vi "Compile APU 1.4 Data.vi"(8 "error in (no error)":errorcluster, 11 "Device Item Ref in":T3 format="%.0x") -> (0 "error out":errorcluster, 2 "APUs":T1[](array[typedef]), 3 "Device Item Ref out":T3 format="%.0x")   [LabVIEW 2015, in "Engine Simulation Toolkit System Explorer.lvlib"]
uses:
  Engine Simulation Toolkit System Explorer.lvlib
  <vilib>/NI Veristand/Custom Device API/Custom Device Item Ref.ctl
  Shared/1.4 APU Engine Data.ctl
  Shared/1.4 APU Engine FIFO Idxs.ctl
  Shared/Properties.vi
  Shared/Constants and GUIDs.vi
  <vilib>/NI Veristand/Custom Device Tools/Custom Device Utility Library/NI VeriStand - Search for All Items by GUID.vi
  <vilib>/NI Veristand/Custom Device API/Get Item Property (String).vi
  <vilib>/NI Veristand/Custom Device API/Get Item Property (Double).vi
  <vilib>/NI Veristand/Custom Device API/Get Item Property (Boolean).vi
  <vilib>/NI Veristand/Custom Device API/Get Item Property (U16).vi
  <vilib>/NI Veristand/Custom Device Tools/Custom Device Utility Library/NI VeriStand - Search for Item by GUID.vi
  Shared/Engine Simulation Toolkit Shared.lvlib
  <vilib>/NI Veristand/Custom Device API/Custom Device API.lvlib
  <vilib>/NI Veristand/Custom Device Tools/Custom Device Utility Library/Custom Device Utility Library.lvlib
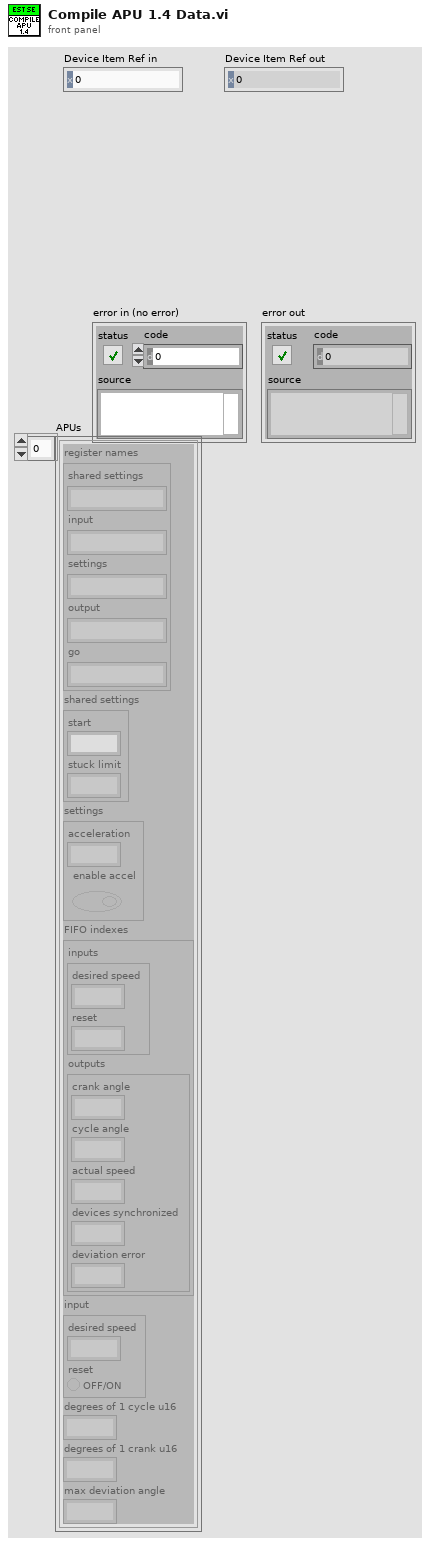
[diagram p1: front panel]
types:
  T1 = typedef "Engine Simulation Toolkit Shared.lvlib/1.4 APU Engine Data.ctl" = cluster{"register names":cluster{"shared settings":string, "input":string, "settings":string, "output":string, "go":string}, "shared settings":cluster{"start":fxp<+,17,17>, "stuck limit":fxp<+,18,18>}, "settings":cluster{"acceleration":fxp<+,18,-20>, "enable accel":bool}, "FIFO indexes":T2, "input":cluster{"desired speed":fxp<+/-,23,2>, "reset":bool}, "degrees of 1 cycle u16":dbl, "degrees of 1 crank u16":dbl, "max deviation angle":dbl}
  T2 = typedef "Engine Simulation Toolkit Shared.lvlib/1.4 APU Engine FIFO Idxs.ctl" = cluster{"inputs":cluster{"desired speed":i32, "reset":i32}, "outputs":cluster{"crank angle":i32, "cycle angle":i32, "actual speed":i32, "devices synchronized":i32, "deviation error":i32}}
  T3 = typedef "Custom Device API.lvlib/Custom Device Item Ref.ctl" = u64
  T4 = typedef "Engine Simulation Toolkit Shared.lvlib/Channel.ctl" = cluster{"Name":string, "Units":string, "Default":dbl, "Description":string, "Scalable":bool}
  T5 = cluster{"desired speed":fxp<+/-,23,2>, "reset":bool}
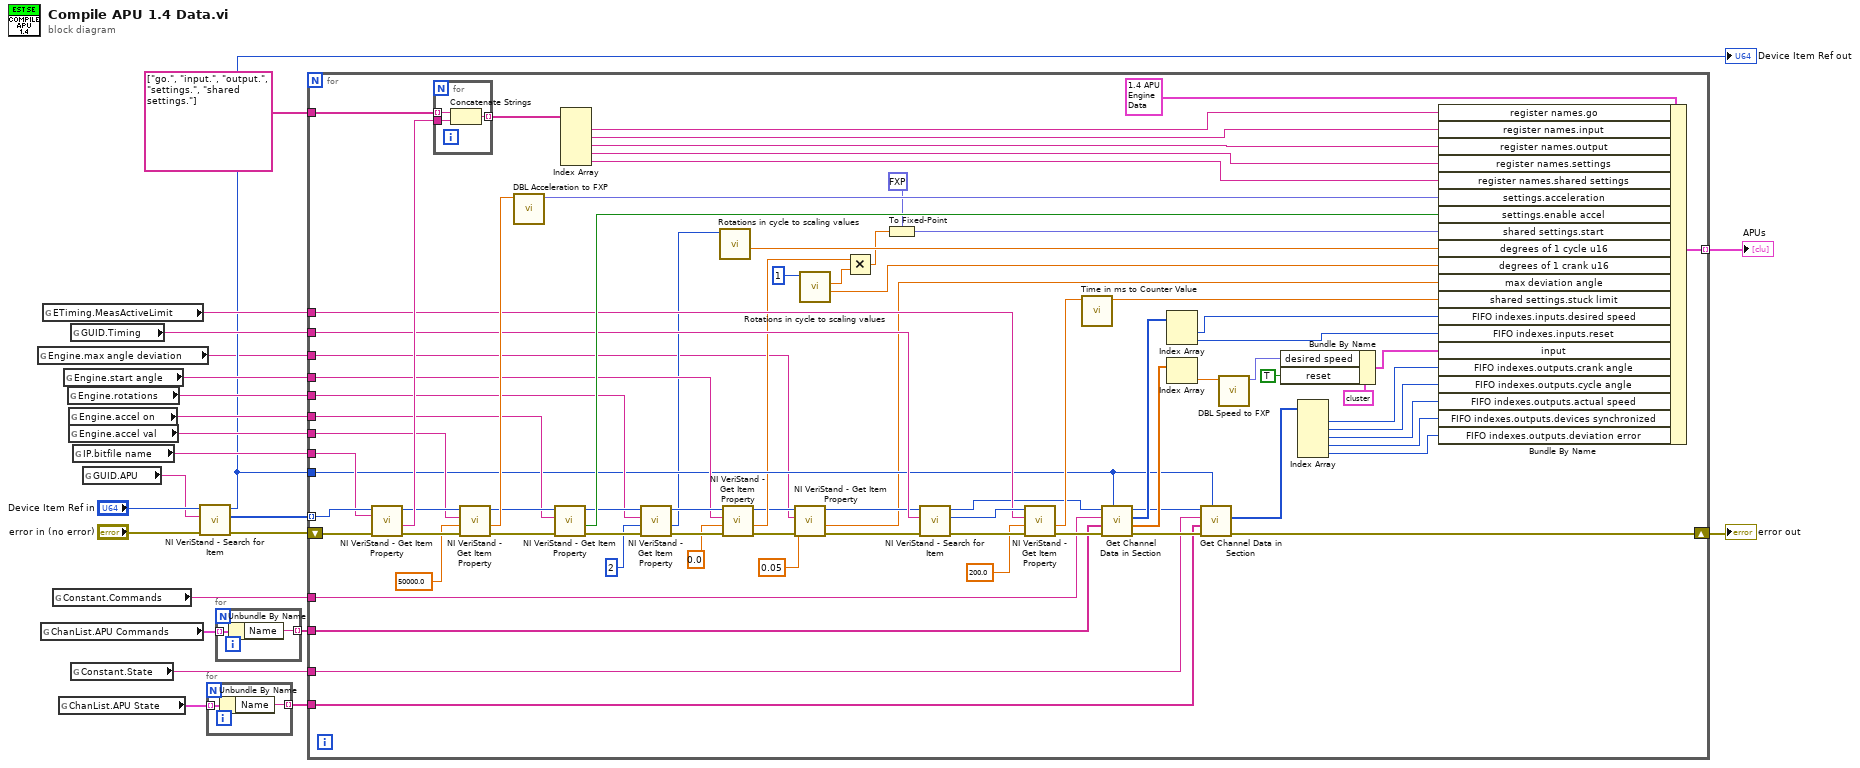
[diagram p0: block diagram]
diagram:
  n1 = global read "Properties.vi" "Engine.max angle deviation"() -> (w1:string)
  n2 = global read "Constants and GUIDs.vi" "ChanList.APU Commands"() -> (w7:T4[])
  n3 = global read "Properties.vi" "ETiming.MeasActiveLimit"() -> (w11:string)
  n4 = global read "Constants and GUIDs.vi" "Constant.Commands"() -> (w10:string)
  n5 = global read "Constants and GUIDs.vi" "ChanList.APU State"() -> (w5:T4[])
  n6 = global read "Properties.vi" "Engine.start angle"() -> (w13:string)
  n7 = global read "Properties.vi" "Engine.rotations"() -> (w14:string)
  n8 = global read "Properties.vi" "Engine.accel on"() -> (w15:string)
  n9 = global read "Properties.vi" "Engine.accel val"() -> (w17:string)
  n10 = global read "Constants and GUIDs.vi" "GUID.Timing"() -> (w12:string)
  n11 = global read "Constants and GUIDs.vi" "Constant.State"() -> (w8:string)
  n12 = global read "Properties.vi" "IP.bitfile name"() -> (w19:string)
  n13 = global read "Constants and GUIDs.vi" "GUID.APU"() -> (w21:string)
  n14 = call-poly <vilib>:"NI VeriStand - Search for Item.vi"("error in"="error in (no error)", "Item GUID"=w21, "Section Ref in"="Device Item Ref in") -> ("error out"=w20:errorcluster, "Item Refs"=w3:T3[], "Section Ref out"=w9:T3)  [unwired: 5 in, 1 out]
  "Device Item Ref out" <- w9
  n15 = for {
    tunnel: w5 -> [w25] mode=indexing
    tunnel: [w24] -> w4 mode=indexing
    n16 = Unbundle By Name(w25) -> ("Name"=w24:string)
  }
  n17 = for {
    tunnel: w7 -> [w27] mode=indexing
    tunnel: [w26] -> w6 mode=indexing
    n18 = Unbundle By Name(w27) -> ("Name"=w26:string)
  }
  n19 = for {
    shift-right: [w62] -> w16
    shift-left: w20 -> [w106]
    tunnel: w3 -> [w105] mode=indexing
    tunnel: w19 -> [w104]
    tunnel: string[] ["go.", "input.", "output.", "settings.", "shared settings."] -> [w102]
    tunnel: w17 -> [w97]
    tunnel: w15 -> [w91]
    tunnel: w14 -> [w87]
    tunnel: w13 -> [w84]
    tunnel: w12 -> [w81]
    tunnel: w11 -> [w78]
    tunnel: w10 -> [w73]
    tunnel: w6 -> [w51]
    tunnel: [w67] -> w2 mode=indexing
    tunnel: w9 -> [w61]
    tunnel: w8 -> [w59]
    tunnel: w4 -> [w50]
    tunnel: w1 -> [w29]
    n20 = call-poly <vilib>:"NI VeriStand - Get Item Property.vi"("error in (no error)"=w106, "Property Name"=w104, "Item Ref in"=w105) -> ("error out"=w98:errorcluster, "Value"=w103:string, "Item Ref out"=w99:T3)  [unwired: 5 in, 1 out]
    n21 = for {
      tunnel: w103 -> [w109]
      tunnel: w102 -> [w108] mode=indexing
      tunnel: [w107] -> w100 mode=indexing
      n22 = Concatenate Strings(w108, w109) -> (w107:string)
    }
    n23 = call-poly <vilib>:"NI VeriStand - Get Item Property.vi"("error in (no error)"=w98, "Default Value"=50000.0, "Property Name"=w97, "Item Ref in"=w99) -> ("error out"=w96:errorcluster, "Value"=w95:dbl, "Item Ref out"=w92:T3)  [unwired: 4 in, 1 out]
    n24 = call "DBL Acceleration to FXP.vi"("Desired acceleration (RPM/sec)"=w95) -> ("FXP acceleration"=w94:fxp<+,18,-20>)  [unwired: 6 in, 4 out]
    n25 = call-poly <vilib>:"NI VeriStand - Get Item Property.vi"("error in (no error)"=w96, "Property Name"=w91, "Item Ref in"=w92) -> ("error out"=w93:errorcluster, "Value"=w90:bool, "Item Ref out"=w88:T3)  [unwired: 5 in, 1 out]
    n26 = Index Array(array=w100) -> (element #1=w49:string, element #2=w48:string, element #3=w47:string, element #4=w46:string, element #5=w45:string)  [unwired: 5 in]
    n27 = call-poly <vilib>:"NI VeriStand - Get Item Property.vi"("error in (no error)"=w93, "Default Value"=u16 2, "Property Name"=w87, "Item Ref in"=w88) -> ("error out"=w89:errorcluster, "Value"=w44:u16, "Item Ref out"=w85:T3)  [unwired: 4 in, 1 out]
    n28 = call "Rotations in cycle to scaling values.vi"("rotations in a cycle"=w44) -> ("degrees of one u16"=w43:dbl)  [unwired: 8 in, 2 out]
    n29 = call-poly <vilib>:"NI VeriStand - Get Item Property.vi"("error in (no error)"=w89, "Default Value"=0.0, "Property Name"=w84, "Item Ref in"=w85) -> ("error out"=w33:errorcluster, "Value"=w41:dbl, "Item Ref out"=w35:T3)  [unwired: 4 in, 1 out]
    n30 = call-poly <vilib>:"NI VeriStand - Get Item Property.vi"("error in (no error)"=w33, "Default Value"=0.05, "Property Name"=w29, "Item Ref in"=w35) -> ("error out"=w32:errorcluster, "Value"=w30:dbl, "Item Ref out"=w31:T3)  [unwired: 4 in, 1 out]
    n31 = call "Rotations in cycle to scaling values.vi"("rotations in a cycle"=u16 1) -> ("degrees of one u16"=w52:dbl, "angle to u16 scale factor"=w42:dbl)  [unwired: 8 in, 1 out]
    n32 = Multiply(x=w41, y=w42) -> (x*y=w40:dbl)
    n33 = To Fixed-Point(fixed-point type=fxp<+,17,17> 0.0 ("shared settings.start"), number=w40) -> (fixed-point=w38:fxp<+,17,17>)
    n34 = call-poly <vilib>:"NI VeriStand - Search for Item.vi"("error in"=w32, "Item GUID"=w81, "Section Ref in"=w31) -> ("error out"=w82:errorcluster, "Item Ref"=w79:T3, "Section Ref out"=w74:T3)  [unwired: 5 in, 1 out]
    n35 = call-poly <vilib>:"NI VeriStand - Get Item Property.vi"("error in (no error)"=w82, "Default Value"=200.0, "Property Name"=w78, "Item Ref in"=w79) -> ("error out"=w80:errorcluster, "Value"=w76:dbl)  [unwired: 4 in, 2 out]
    n36 = call "Time in ms to Counter Value.vi"("time (ms)"=w76) -> ("counter value"=w75:dbl)  [unwired: 10 in]
    n37 = call "Get Channel Data in Section.vi"("Custom device ref"=w61, "error in (no error)"=w80, "Channels"=w51, "Section (\"\":none)"=w73, "Item Ref in"=w74) -> ("error out"=w72:errorcluster, "default values"=w66:dbl[], "FIFO indexes"=w71:i32[], "Item Ref out"=w60:T3)  [unwired: 2 in, 1 out]
    n38 = Index Array(array=w71) -> (element #1=w70:i32, element #2=w69:i32)  [unwired: 2 in]
    n39 = Index Array(array=w66) -> (element=w65:dbl)  [unwired: 1 in]
    n40 = call "Get Channel Data in Section.vi"("Custom device ref"=w61, "error in (no error)"=w72, "Channels"=w50, "Section (\"\":none)"=w59, "Item Ref in"=w60) -> ("error out"=w62:errorcluster, "FIFO indexes"=w58:i32[])  [unwired: 2 in, 3 out]
    n41 = call "DBL Speed to FXP.vi"("Desired speed (RPM)"=w65) -> ("FXP speed"=w63:fxp<+/-,23,2>)  [unwired: 6 in, 4 out]
    n42 = Bundle By Name(cluster=T5 {"desired speed"=0.0, "reset"=FALSE} ("input"), "desired speed"=w63, "reset"=TRUE) -> (w64:T5)
    n43 = Index Array(array=w58) -> (element #1=w57:i32, element #2=w56:i32, element #3=w55:i32, element #4=w36:i32, element #5=w37:i32)  [unwired: 5 in]
    n44 = Bundle By Name(cluster=T1 {"register names"={"shared settings"="", "input"="", "settings"="", "output"="", "go"=""}, "shared settings"={"start"=0.0, "stuck limit"=0.0}, "settings"={"acceleration"=0.0, "enable accel"=FALSE}, "FIFO indexes"={"inputs"={"desired speed"=0, "reset"=0}, "outputs"={"crank angle"=0, "cycle angle"=0, "actual speed"=0, "devices synchronized"=0, "deviation error"=0}}, "input"={"desired speed"=0.0, "reset"=FALSE}, "degrees of 1 cycle u16"=0.0, "degrees of 1 crank u16"=0.0, "max deviation angle"=0.0} ("1.0.0 APU"), "register names.go"=w49, "register names.input"=w48, "register names.output"=w47, "register names.settings"=w46, "register names.shared settings"=w45, "settings.acceleration"=w94, "settings.enable accel"=w90, "shared settings.start"=w38, "degrees of 1 cycle u16"=w43, "degrees of 1 crank u16"=w52, "max deviation angle"=w30, "shared settings.stuck limit"=w75, "FIFO indexes.inputs.desired speed"=w70, "FIFO indexes.inputs.reset"=w69, "input"=w64, "FIFO indexes.outputs.crank angle"=w57, "FIFO indexes.outputs.cycle angle"=w56, "FIFO indexes.outputs.actual speed"=w55, "FIFO indexes.outputs.devices synchronized"=w36, "FIFO indexes.outputs.deviation error"=w37) -> (w67:T1)
  }
  "error out" <- w16
  "APUs" <- w2
